vi "WebCam Grab_FLIR_trig.vi"(0 "Session In":T3, 1 "Image In":T2, 2 "Buffer Number In":u32, 3 "Trial Time":dbl, 4 "AVI Refnum":T1, 5 "error in":errorcluster) -> (14 "Session Out":T3, 15 "WebCam Img Out":T2, 17 "Buffer Number Out":u32, 19 "error out":errorcluster)   [LabVIEW 2020]
uses:
  <vilib>/userDefined/High Color/IMAQdx.ctl
  <vilib>/vision/Image Controls.llb/IMAQ Image.ctl
  <vilib>/vision/Avi.llb/IMAQ AVI2 Refnum.ctl
  <vilib>/vision/driver/IMAQdx.llb/IMAQdx Buffer Number Mode.ctl
  <vilib>/vision/NI_Vision_Development_Module.lvlib
  <vilib>/vision/driver/NI_Vision_Acquisition_Software.lvlib
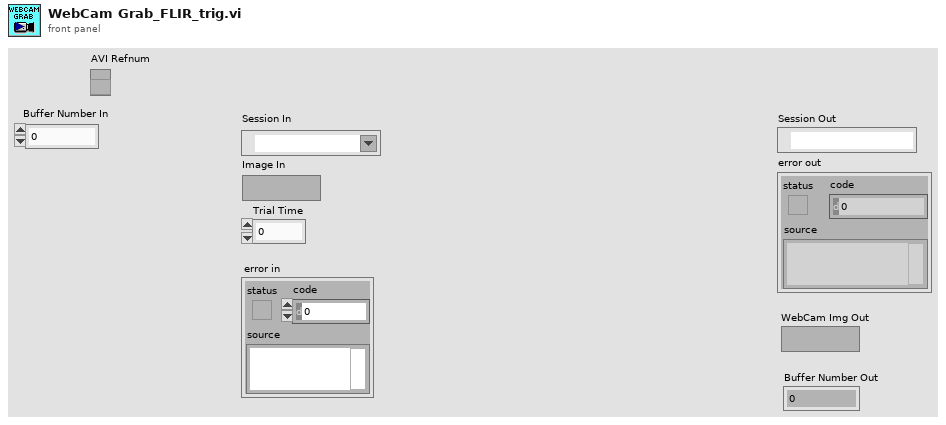
[diagram p1: front panel]
types:
  T1 = typedef "IMAQ AVI2 Refnum.ctl" = refnum<k20>
  T2 = typedef "IMAQ Image.ctl" = refnum<image>
  T3 = typedef "IMAQdx.ctl" = refnum<k21>
  T4 = typedef "NI_Vision_Acquisition_Software.lvlib/IMAQdx Buffer Number Mode.ctl" = enum32{"Next", "Last", "Buffer Number", "Every", "Last New"}
  T5 = cluster{"Desired Font (Application)":enum16{"User-specified Font", "Application Font", "System Font", "Dialog Font"}, "[User-specified Font]":cluster{"Font Name":string, "Size":i16, "Strikeout?":bool, "Italic?":bool, "Underline?":bool, "Outline?":bool, "Shadow?":bool, "Bold?":bool, "Rotation Angle":dbl}, "Horizontal Alignment":i16, "Vertical Alignment":i16}
  T6 = typedef "Image Type" = u32
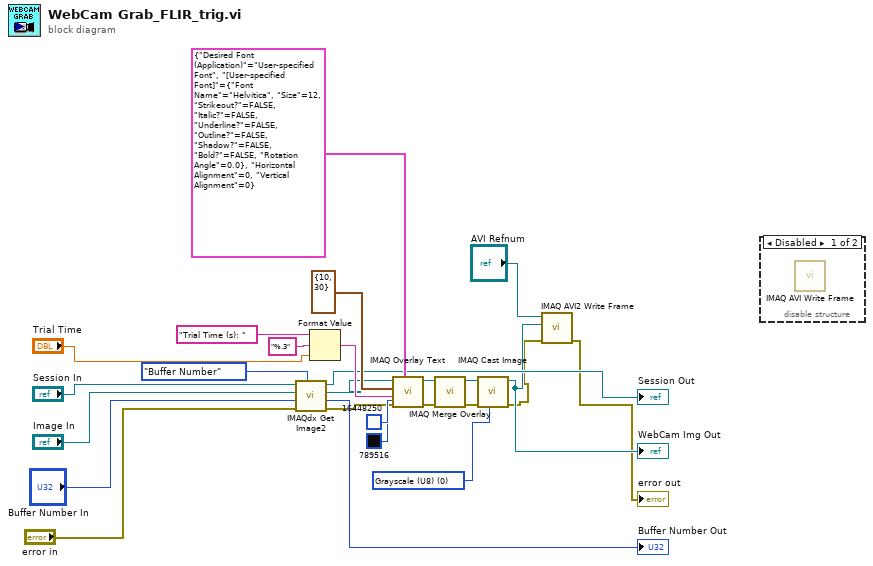
[diagram p0: block diagram]
diagram:
  w26 = T6 0 items=["Grayscale (U8)", "Grayscale (I16)", "Grayscale (SGL)", "Complex (CSG)", "RGB (U32)", "HSL (U32)", "RGB (U64)", "Grayscale (U16)"] ("Image Type")
  n1 = call <vilib>:"IMAQdx Get Image2.vi"("Buffer Number Mode (Next)"=IMAQdx_Buffer_Number_Mode."Buffer Number", "error in"="error in", "Buffer Number In"="Buffer Number In", "Image In"="Image In", "Session In"="Session In") -> ("error out"=w5:errorcluster, "Buffer Number Out"=→"Buffer Number Out":u32, "Image Out"=w7:T2, "Session Out"=→"Session Out":T3)  [unwired: 3 in]
  n2 = Format Value(string ("")="Trial Time (s): ", format string="%.3", value (0)="Trial Time") -> (output string=w17:string)
  n3 = call "IMAQ Overlay Text"("BG Color (Transparent)"=u32 789516, "Text Color (black)"=u32 16448250, "Font, Size & Style"=T5 {"Desired Font (Application)"=enum."User-specified Font", "[User-specified Font]"={"Font Name"="Helvitica", "Size"=12, "Strikeout?"=FALSE, "Italic?"=FALSE, "Underline?"=FALSE, "Outline?"=FALSE, "Shadow?"=FALSE, "Bold?"=FALSE, "Rotation Angle"=0.0}, "Horizontal Alignment"=0, "Vertical Alignment"=0}, "error in (no error)"=w5, "String"=w17, "Origin"=cluster{"X":i32, "Y":i32} {"X"=10, "Y"=30}, "Image"=w7) -> ("error out"=w20:errorcluster, "Image Out"=w21:T2)  [unwired: 3 in]
  n4 = call "IMAQ Merge Overlay"("error in (no error)"=w20, "Image Src"=w21) -> ("error out"=w18:errorcluster, "Image Dst Out"=w19:T2)  [unwired: 8 in]
  n5 = call "IMAQ Cast Image"("Image Type"=w26, "error in (no error)"=w18, "Image Src"=w19) -> ("error out"=w3:errorcluster, "Image Dst Out"=w4:T2)  [unwired: 7 in]
  "WebCam Img Out" <- w4
  n6 = call "IMAQ AVI2 Write Frame"("error in (no error)"=w3, "Image"=w4, "AVI Refnum"="AVI Refnum") -> ("error out"=→"error out":errorcluster)  [unwired: 6 in, 2 out]
  n7 = disable-structure shown="Disabled" {
    frame Disabled {
      n8 = call "IMAQ AVI Write Frame"() -> ()  [unwired: 10 in, 2 out]
    }
    frame Enabled {
    }
  }
